vi "Set color of CMD buttons.vi"(6 "Color OFF":u32(colorbox)=32832, 7 "Color ON":u32(colorbox)=7204608, 8 "error in (no error)":errorcluster, 9 "Var Index":i32, 10 "Values":T1[](array[typedef]), 11 "Ctrl ref":refnum<vi>) -> (0 "error out":errorcluster)   [LabVIEW 2011]
uses:
  Measurments Handling/Status Digitalish.ctl
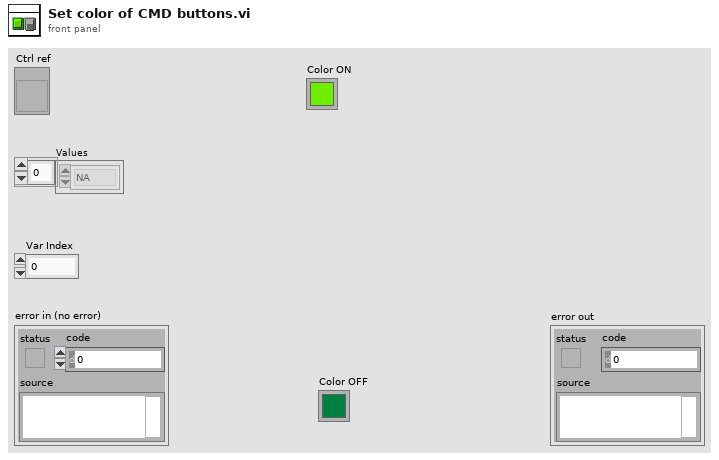
[diagram p1: front panel]
types:
  T1 = typedef "Status Digitalish.ctl" = enum16{"NA", "False", "True"}
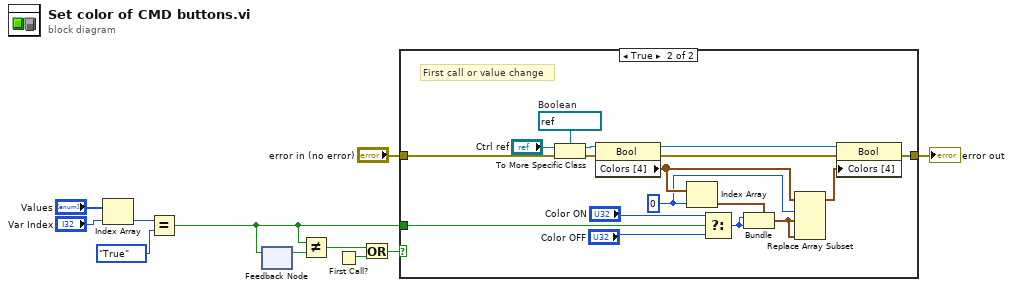
[diagram p0: block diagram]
diagram:
  n1 = Index Array(array="Values", index="Var Index") -> (element=w3:T1)
  n2 = Equal?(x=w3, y=Status_Digitalish."True" ("element")) -> (x = y?=w4:bool)
  n3 = feedback-in #1(w4) -> ()
  n4 = feedback #1() -> (w9:bool)  [unwired: 1 in]
  n5 = Not Equal?(x=w4, y=w9) -> (x != y?=w7:bool)
  n6 = First Call?() -> (First Call?: T/F=w8:bool)
  n7 = Or(x=w7, y=w8) -> (x .or. y?=w6:bool)
  n8 = case shown="True" w6 {
    tunnel: "error in (no error)" -> [w12 w19]
    tunnel: [w12 w14] -> w10
    tunnel: w4 -> [_ w17]
    frame False {
    }
    frame True {
      w26 = refnum<vi> refnum  # Boolean
      w22 = 0 ("index")
      # "First call or value change"
      n9 = To More Specific Class(target class=w26, reference="Ctrl ref", error in=w19) -> (specific class reference=w25:refnum<vi>, error out=w28:errorcluster)
      n10 = property on="Property Node" class="Bool"(reference=w25, error in=w28) -> (reference out=w27:refnum<vi>, error out=w29:errorcluster, "Colors [4]"=w23:cluster{u32, u32}[])
      n11 = Index Array(array=w23, index=w22) -> (element=w24:cluster{u32, u32})
      n12 = Select(t="Color ON", s=w17, f="Color OFF") -> (s? t:f=w16:u32)
      n13 = Bundle(cluster=w24, w16, w16) -> (w13:cluster{u32, u32})
      n14 = Replace Array Subset(array=w23, new element #1=w13, index #1=w22, new element #2=w13) -> (w21:cluster{u32, u32}[])  [unwired: 1 in]
      n15 = property on="Property Node" class="Bool"(reference=w27, error in=w29, "Colors [4]"=w21) -> (error out=w14:errorcluster)  [unwired: 1 out]
    }
  }
  "error out" <- w10
